vi "disconnect.vi"(8 "error in (no error)":errorcluster, 11 "connection ID":refnum<k5>) -> (0 "error out":errorcluster)   [LabVIEW 2010]
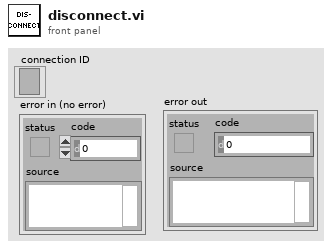
[diagram p1: front panel]
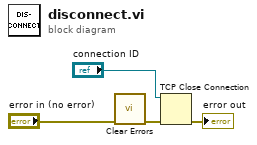
[diagram p0: block diagram]
diagram:
  n1 = call <vilib>:"Clear Errors.vi"("error in (no error)"="error in (no error)") -> ("error out"=w4:errorcluster)  [unwired: 6 in]
  n2 = TCP Close Connection(connection ID="connection ID", error in (no error)=w4) -> (error out=→"error out":errorcluster)  [unwired: 1 in, 1 out]
